vi "ScaledWaveform-UpdateWaveforms.vi"(8 "Error in":errorcluster, 11 "Custom Device ref in":T1 format="%.0x") -> (0 "Error out":errorcluster, 3 "Custom Device ref out":T1=18446744073709551615 format="%.0x")   [LabVIEW 2015, in "Waveform-Processing-Custom-Device Shared.lvlib" / "Scaled Waveform.lvlib"]
uses:
  Scaled Waveform.lvlib
  <vilib>/NI VeriStand/Custom Device API/Custom Device API.lvlib
  <vilib>/NI Veristand/Custom Device API/Get Item Property (Boolean).vi
  Constants.vi
  Waveform-Processing-Custom-Device Shared.lvlib
  <vilib>/NI Veristand/Custom Device API/Custom Device Item Ref.ctl
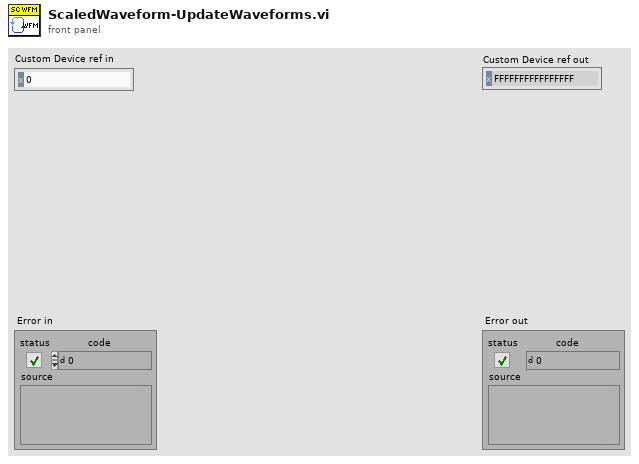
[diagram p1: front panel]
types:
  T1 = typedef "Custom Device API.lvlib/Custom Device Item Ref.ctl" = u64
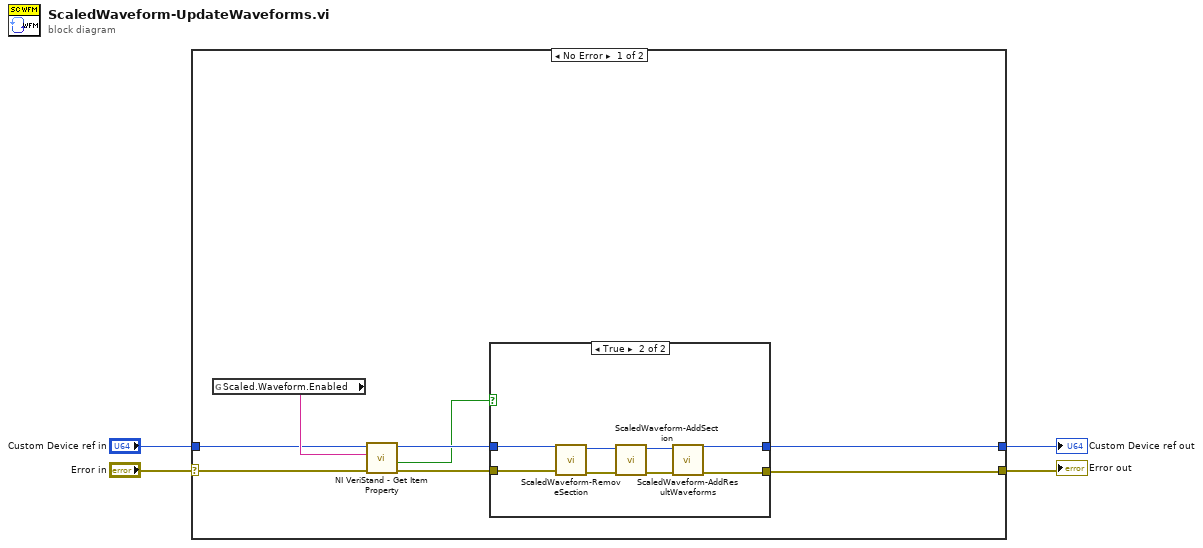
[diagram p0: block diagram]
diagram:
  n1 = case shown="No Error" "Error in" {
    selector: "Error in" -> [w5 w24]
    tunnel: [w12 w24] -> w3
    tunnel: "Custom Device ref in" -> [w6 w23]
    tunnel: [w11 w23] -> w1
    frame No Error {
      n2 = global read "Constants.vi" "Scaled.Waveform.Enabled"() -> (w9:string)
      n3 = call-poly <vilib>:"NI VeriStand - Get Item Property.vi"("error in (no error)"=w5, "Property Name"=w9, "Item Ref in"=w6) -> ("error out"=w10:errorcluster, "Value"=w7:bool, "Item Ref out"=w8:T1)  [unwired: 5 in, 1 out]
      n4 = case shown="True" w7 {
        tunnel: w10 -> [w13 w20]
        tunnel: [w13 w22] -> w12
        tunnel: w8 -> [w14 w19]
        tunnel: [w14 w21] -> w11
        frame False {
        }
        frame True {
          n5 = call "ScaledWaveform-RemoveSection.vi"("Error in"=w20, "Custom Device ref"=w19) -> ("Error out"=w16:errorcluster, "Custom Device ref out"=w18:T1)  [unwired: 8 in]
          n6 = call "ScaledWaveform-AddSection.vi"("Error in"=w16, "Custom Device ref"=w18) -> ("Error out"=w15:errorcluster, "Custom Device ref out"=w17:T1)  [unwired: 8 in]
          n7 = call "ScaledWaveform-AddResultWaveforms.vi"("Error in"=w15, "Custom Device ref"=w17) -> ("Error out"=w22:errorcluster, "Custom Device ref out"=w21:T1)  [unwired: 8 in]
        }
      }
    }
    frame Error {
    }
  }
  "Error out" <- w3
  "Custom Device ref out" <- w1
